vi "Get configuration chain.vi"(8 "error in (no error)":errorcluster, 11 "TemplateBase in":refnum<class "Cobolt.lvclass">=refnum) -> (0 "error out":errorcluster, 1 "class name":string[](array[string]), 2 "configuration chain":variant[](array[variant]), 3 "TemplateBase out":refnum<class "Cobolt.lvclass">)   [LabVIEW 2012, in "Cobolt.lvclass"]
doc: "Returns an array of variants containing the configuration clusters of each class in the inheritance chain (lowest child class first), together with an array of all class names in the inheritance chain.\n\nFor classes without configuration cluster, the configuration chain contains empty variants."
uses:
  Cobolt.lvclass
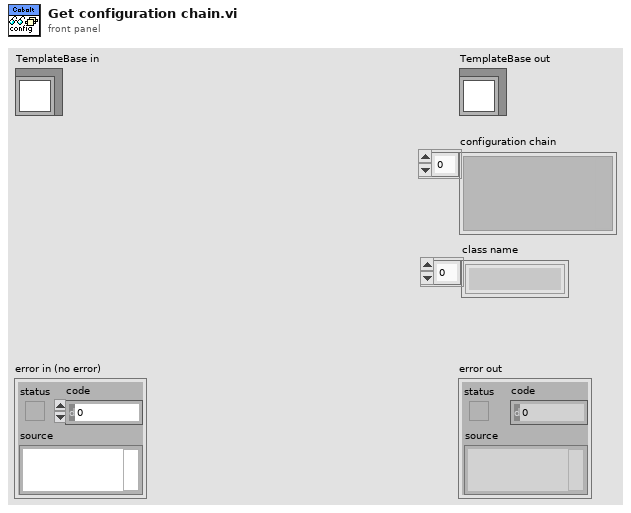
[diagram p1: front panel]
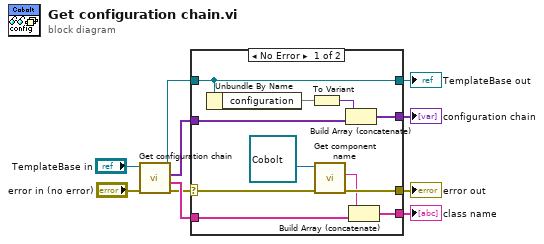
[diagram p0: block diagram]
diagram:
  n1 = call-parent "Get configuration chain.vi"("error in (no error)"="error in (no error)", "MurmexBase in"="TemplateBase in") -> ("error out"=w4:errorcluster, "class name"=w5:string[], "configuration chain"=w7:variant[], "MurmexBase out"=w2:refnum<class "Cobolt.lvclass">)  [unwired: 6 in]
  n2 = case shown="No Error" w4 {
    selector: w4 -> [w18 w23]
    tunnel: [w17 w23] -> w3
    tunnel: [w14 w22] -> w1
    tunnel: w2 -> [w14 w22]
    tunnel: [w19 _] -> w6
    tunnel: [w15 _] -> w8
    tunnel: w7 -> [w13 _]
    tunnel: w5 -> [w12 _]
    frame No Error {
      n3 = Unbundle By Name(w14) -> ("configuration"=w21)
      n4 = To Variant(anything=w21) -> (Variant=w20:variant)
      n5 = call "Get component name.vi"("error in (no error)"=w18, "Murmex in"=refnum<class "Cobolt.lvclass"> refnum ("Template.lvclass")) -> ("error out"=w17:errorcluster, "component name"=w16:string)  [unwired: 7 in, 1 out]
      n6 = Build Array (concatenate)(w20, w13) -> (w19:variant[])
      n7 = Build Array (concatenate)(w16, w12) -> (w15:string[])
    }
    frame Error {
    }
  }
  "error out" <- w3
  "TemplateBase out" <- w1
  "configuration chain" <- w6
  "class name" <- w8
